vi "Flasher.vi"(5 "reference":refnum<vi>) -> ()   [LabVIEW 2020]
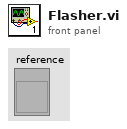
[diagram p1: front panel]
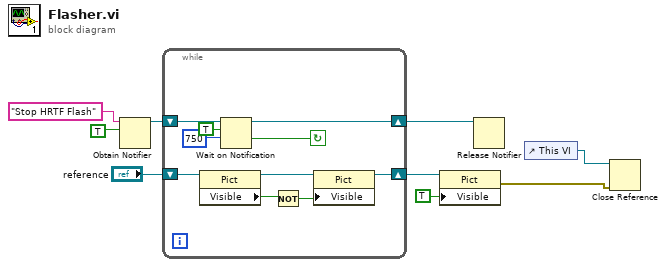
[diagram p0: block diagram]
diagram:
  n1 = Obtain Notifier(name (unnamed)="Stop HRTF Flash", notification data type=TRUE) -> (notifier out=w6:refnum<notifier>)  [unwired: 2 in, 2 out]
  n2 = while {
    shift-right: [w13] -> w5
    shift-left: w6 -> [w15]
    shift-right: [w10] -> w4
    shift-left: "reference" -> [w16]
    stop <- w12 continue-if-true
    n3 = property class="Pict"(reference=w16) -> (reference out=w19:refnum<vi>, "Visible"=w18:bool)  [unwired: 1 in, 1 out]
    n4 = Wait on Notification(notifier=w15, ignore previous (F)=TRUE, timeout in ms (-1)=u32 750 ("milliseconds to wait")) -> (notifier out=w13:refnum<notifier>, timed out?=w12:bool)  [unwired: 1 in, 2 out]
    n5 = Not(x=w18) -> (.not. x?=w17:bool)
    n6 = property class="Pict"(reference=w19, "Visible"=w17) -> (reference out=w10:refnum<vi>)  [unwired: 1 in, 1 out]
  }
  n7 = property class="Pict"(reference=w4, "Visible"=TRUE) -> (error out=w1:errorcluster)  [unwired: 1 in, 1 out]
  n8 = Release Notifier(notifier=w5) -> ()  [unwired: 2 in, 3 out]
  n9 = control-ref of="This VI"() -> (w2:refnum<vi>)
  n10 = Close Reference(reference=w2, error in (no error)=w1) -> ()  [unwired: 1 out]
